vi "Gill_parse_response.vi"(0 "Address letter":string, 1 "Stripped Gill response":string, 2 "GILL TYPE NO.":i32) -> (4 "Numerics":dbl[](array[numeric]) format="%.2f", 5 "Status":u8, 6 "Error notes":string)   [LabVIEW 2010]
panel:
  out "Type\nModel 2":u8
  out "Type\nModel":u8
  in  "Status Messages":string[](array[string])=["", "Transducer Pair 1 failed", "Transducer Pair 2 failed", "Transducers 1 & 2 failed", "Non-volatile Checksum error", "Volatile memory checksum error", "System gain at maximum", "Marginal system gain condition", "Measurement average building", "Heating operational", "Heating OK but under power", "Heating tripped", "Temperature sensor fault", "Heating OK but over power"]
  in  "Status Codes":u8[](array[numeric])=[0, 1, 2, 4, 8, 9, 10, 50, 51, 60, 61, 62, 63, 64]
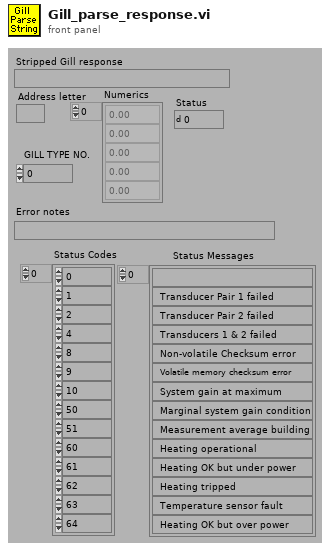
[diagram p1: front panel]
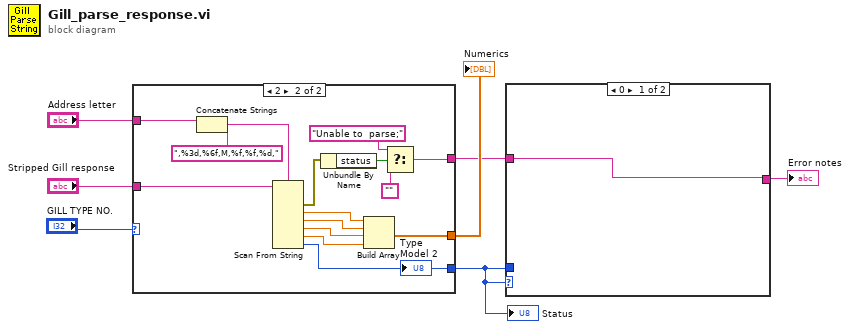
[diagram p0: block diagram]
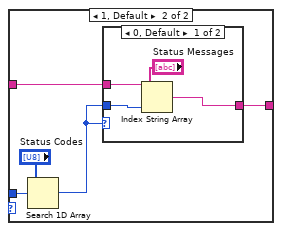
[diagram p2: hidden frame]
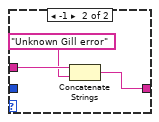
[diagram p3: hidden frame]
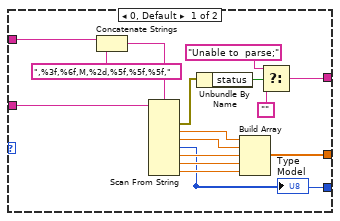
[diagram p4: hidden frame]
diagram:
  n1 = case shown="2" "GILL TYPE NO." {
    tunnel: "Stripped Gill response" -> [w23 w38]
    tunnel: "Address letter" -> [w22 w37]
    tunnel: [w15 w34] -> w5
    tunnel: [w10 w29] -> w3
    tunnel: [w8 w24] -> w1
    frame 0, Default {
      n2 = Concatenate Strings(w22, ",%3f,%6f,M,%2d,%5f,%5f,%5f,") -> (w21:string)
      n3 = Scan From String(format string=w21, input string=w23) -> (error out=w13:errorcluster, output 1=w16:dbl, output 2=w17:dbl, output 3=w8:u8, output 4=w18:dbl, output 5=w19:dbl, output 6=w20:dbl)  [unwired: 2 in, 8 out]
      "Type\nModel" <- w8
      n4 = Unbundle By Name(w13) -> ("status"=w12:bool)
      n5 = Build Array(w16, w17, w18, w19, w20) -> (w15:dbl[])
      n6 = Select(t="Unable to  parse;", s=w12, f="") -> (s? t:f=w10:string)
    }
    frame 2 {
      n7 = Concatenate Strings(w37, ",%3d,%6f,M,%f,%f,%d,") -> (w25:string)
      n8 = Scan From String(format string=w25, input string=w38) -> (error out=w32:errorcluster, output 1=w35:dbl, output 2=w36:dbl, output 3=w27:dbl, output 4=w26:dbl, output 5=w24:u8)  [unwired: 2 in, 7 out]
      "Type\nModel 2" <- w24
      n9 = Unbundle By Name(w32) -> ("status"=w31:bool)
      n10 = Build Array(w35, w36, w27, w26) -> (w34:dbl[])
      n11 = Select(t="Unable to  parse;", s=w31, f="") -> (s? t:f=w29:string)
    }
  }
  "Numerics" <- w5
  "Status" <- w1
  n12 = case shown="0" w1 {
    tunnel: w1 -> [_ w43]
    tunnel: w3 -> [w39 w42]
    tunnel: [w39 w41] -> w2
    frame 0 {
    }
    frame 1, Default {
      n13 = Search 1D Array(1D array="Status Codes", element=w43) -> (index of element=w40:i32)  [unwired: 1 out]
      n14 = case shown="0, Default" w40 {
        tunnel: w42 -> [w48 w51]
        tunnel: [w47 w50] -> w41
        tunnel: w40 -> [w45 _]
        frame 0, Default {
          n15 = Index String Array(1:w45, 2:"Status Messages", 3:w48) -> (0:w47:string)
        }
        frame -1 {
          n16 = Concatenate Strings(w51, "Unknown Gill error" ("Substring")) -> (w50:string)
        }
      }
    }
  }
  "Error notes" <- w2
